vi "Close.vi"(8 "error in (no error)":errorcluster, 11 "Data in":refnum<class "Fault-Injection Bus.lvclass">) -> (0 "error out":errorcluster, 3 "Data out":refnum<class "Fault-Injection Bus.lvclass">)   [LabVIEW 2021, in "Fault-Injection Bus.lvclass"]
doc: "Abstract Data Classes 2.1.1.12\nTim Streeter - TSA\nCopyright (c) 2024, TSA"
uses:
  Fault-Injection Bus.lvclass
  Fault-Injection Bus.lvclass/Fault-Injection Bus.ctl
  Properties/Read Buses.vi
  Properties/Read Data DVR.vi
  Properties/Read Arm.vi
  Omni-Bus/Bus Access/Bus_Access.lvclass
  <vilib>/TSA/Abstract Data Classes/Abs_Types/Boolean/Abs_Boolean.lvclass
  <vilib>/TSA/Abstract Data Classes/Abs_Types/Single Float/Abs_Single Float.lvclass
  <vilib>/TSA/Abstract Data Classes/Abs_Types/Extended Float/Abs_Extended Float.lvclass
  <vilib>/TSA/Abstract Data Classes/Abs_Types/Type/Abs_Type.lvclass
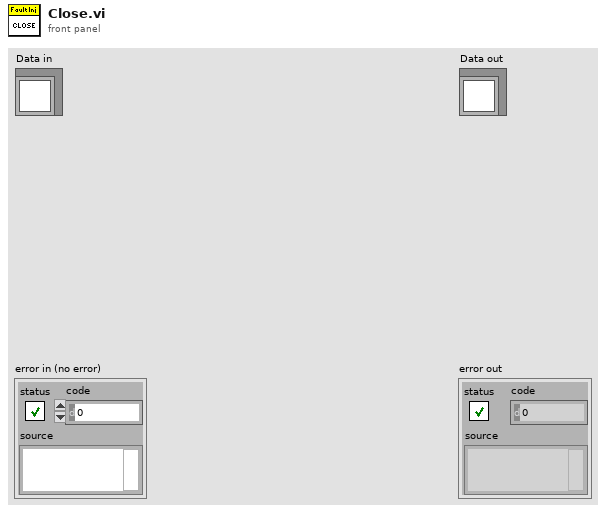
[diagram p1: front panel]
types:
  T1 = typedef "Fault-Injection Bus.lvclass/DVR Type.ctl" = cluster{"Boolean":refnum<data-value>, "String":refnum<data-value>, "DBL":refnum<data-value>, "SGL":refnum<data-value>, "EXT":refnum<data-value>, "U8":refnum<data-value>, "U16":refnum<data-value>, "U32":refnum<data-value>, "U64":refnum<data-value>, "I8":refnum<data-value>, "I16":refnum<data-value>, "I32":refnum<data-value>, "I64":refnum<data-value>, "CDBL":refnum<data-value>, "CSGL":refnum<data-value>, "CEXT":refnum<data-value>, "Time":refnum<data-value>, "Variant":refnum<data-value>, "Waveform":refnum<data-value>, "Type":refnum<data-value>}
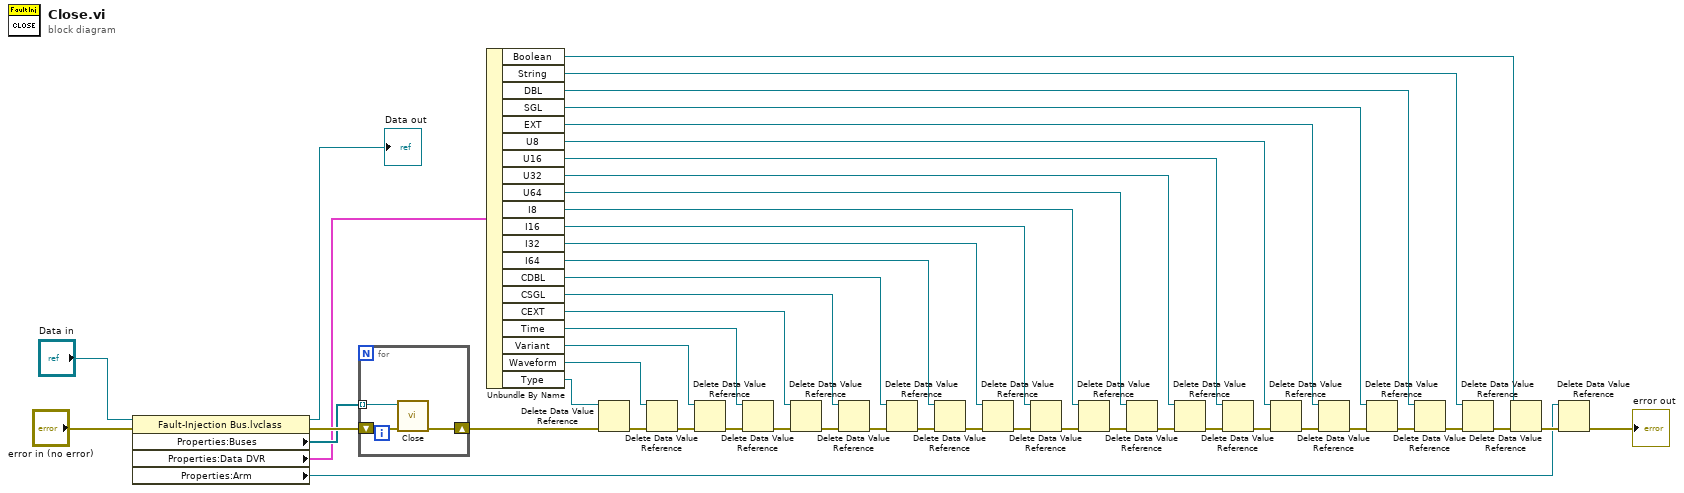
[diagram p0: block diagram]
diagram:
  n1 = property class="Fault-Injection Bus.lvclass"(reference="Data in", error in="error in (no error)") -> (reference out=→"Data out":refnum<class "Fault-Injection Bus.lvclass">, error out=w47:errorcluster, "Properties:Buses"=w46:refnum<class "Bus_Access.lvclass">[], "Properties:Data DVR"=w45:T1, "Properties:Arm"=w3:refnum<data-value>)
  n2 = for {
    shift-right: [w50] -> w44
    shift-left: w47 -> [w52]
    tunnel: w46 -> [w51] mode=indexing
    n3 = call-dynamic "Close.vi"("error in (no error)"=w52, "Data in"=w51) -> ("error out"=w50:errorcluster)  [unwired: 8 in, 1 out]
  }
  n4 = Unbundle By Name(w45) -> ("Boolean"=w5:refnum<data-value>, "String"=w6:refnum<data-value>, "DBL"=w7:refnum<data-value>, "SGL"=w8:refnum<data-value>, "EXT"=w9:refnum<data-value>, "U8"=w10:refnum<data-value>, "U16"=w17:refnum<data-value>, "U32"=w18:refnum<data-value>, "U64"=w19:refnum<data-value>, "I8"=w20:refnum<data-value>, "I16"=w21:refnum<data-value>, "I32"=w27:refnum<data-value>, "I64"=w28:refnum<data-value>, "CDBL"=w29:refnum<data-value>, "CSGL"=w30:refnum<data-value>, "CEXT"=w31:refnum<data-value>, "Time"=w32:refnum<data-value>, "Variant"=w33:refnum<data-value>, "Waveform"=w34:refnum<data-value>, "Type"=w35:refnum<data-value>)
  n5 = Delete Data Value Reference(data value reference=w35, error in=w44) -> (error out=w43:errorcluster)  [unwired: 1 out]
  n6 = Delete Data Value Reference(data value reference=w34, error in=w43) -> (error out=w42:errorcluster)  [unwired: 1 out]
  n7 = Delete Data Value Reference(data value reference=w33, error in=w42) -> (error out=w41:errorcluster)  [unwired: 1 out]
  n8 = Delete Data Value Reference(data value reference=w32, error in=w41) -> (error out=w40:errorcluster)  [unwired: 1 out]
  n9 = Delete Data Value Reference(data value reference=w31, error in=w40) -> (error out=w39:errorcluster)  [unwired: 1 out]
  n10 = Delete Data Value Reference(data value reference=w30, error in=w39) -> (error out=w38:errorcluster)  [unwired: 1 out]
  n11 = Delete Data Value Reference(data value reference=w29, error in=w38) -> (error out=w37:errorcluster)  [unwired: 1 out]
  n12 = Delete Data Value Reference(data value reference=w28, error in=w37) -> (error out=w36:errorcluster)  [unwired: 1 out]
  n13 = Delete Data Value Reference(data value reference=w27, error in=w36) -> (error out=w26:errorcluster)  [unwired: 1 out]
  n14 = Delete Data Value Reference(data value reference=w21, error in=w26) -> (error out=w25:errorcluster)  [unwired: 1 out]
  n15 = Delete Data Value Reference(data value reference=w20, error in=w25) -> (error out=w24:errorcluster)  [unwired: 1 out]
  n16 = Delete Data Value Reference(data value reference=w19, error in=w24) -> (error out=w23:errorcluster)  [unwired: 1 out]
  n17 = Delete Data Value Reference(data value reference=w18, error in=w23) -> (error out=w22:errorcluster)  [unwired: 1 out]
  n18 = Delete Data Value Reference(data value reference=w17, error in=w22) -> (error out=w16:errorcluster)  [unwired: 1 out]
  n19 = Delete Data Value Reference(data value reference=w10, error in=w16) -> (error out=w15:errorcluster)  [unwired: 1 out]
  n20 = Delete Data Value Reference(data value reference=w9, error in=w15) -> (error out=w11:errorcluster)  [unwired: 1 out]
  n21 = Delete Data Value Reference(data value reference=w8, error in=w11) -> (error out=w12:errorcluster)  [unwired: 1 out]
  n22 = Delete Data Value Reference(data value reference=w7, error in=w12) -> (error out=w13:errorcluster)  [unwired: 1 out]
  n23 = Delete Data Value Reference(data value reference=w6, error in=w13) -> (error out=w14:errorcluster)  [unwired: 1 out]
  n24 = Delete Data Value Reference(data value reference=w5, error in=w14) -> (error out=w4:errorcluster)  [unwired: 1 out]
  n25 = Delete Data Value Reference(data value reference=w3, error in=w4) -> (error out=→"error out":errorcluster)  [unwired: 1 out]
